vi "assemblies to tables.vi"(11 "assemblies":T1[](array[typedef])) -> (3 "Item Names":string[][](array[string]))   [LabVIEW 2013, in "EthernetIP editor node.lvclass"]
uses:
  EthernetIP editor node.lvclass
  configuration/assembly type.ctl
  configuration/EthernetIP configuration.lvclass
  configuration/assembly definition.ctl
  <vilib>/NI/Tag Bus/tag/Data Type.ctl
  <vilib>/NI/Tag Bus/tag/tag descriptor.lvclass
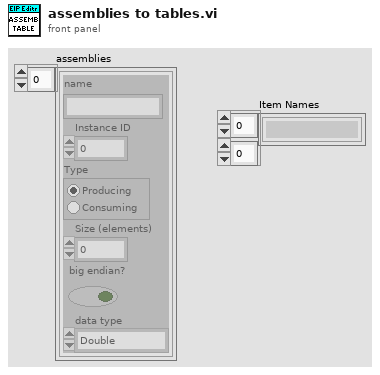
[diagram p1: front panel]
types:
  T1 = typedef "EthernetIP configuration.lvclass/assembly definition.ctl" = cluster{"name":string, "Instance ID":u32, "Type":T2, "Size (elements)":u32, "big endian?":bool, "data type":T3}
  T2 = typedef "EthernetIP configuration.lvclass/assembly type.ctl" = enum32{"Producing", "Consuming"}
  T3 = typedef "tag bus.lvlib/tag descriptor.lvclass/Data Type.ctl" = enum16{"Double", "Single", "I64", "I32", "I16", "I8", "U64", "U32", "U16", "U8", "Boolean", "String", "Array of Double", "Array of Single", "Array of I64", "Array of I32", "Array of I16", "Array of I8", "Array of U64", "Array of U32", "Array of U16", "Array of U8", "Array of Boolean", "Array of String"}
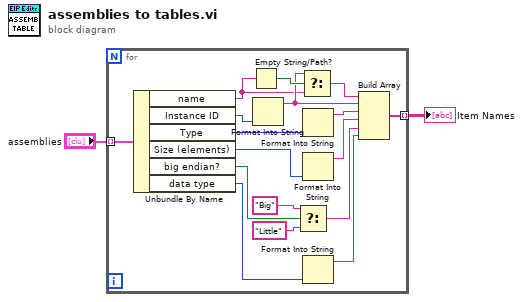
[diagram p0: block diagram]
diagram:
  n1 = for {
    tunnel: "assemblies" -> [w19] mode=indexing
    tunnel: [w13] -> w1 mode=indexing
    n2 = Unbundle By Name(w19) -> ("name"=w9:string, "Instance ID"=w16:u32, "Type"=w17:T2, "Size (elements)"=w18:u32, "big endian?"=w6:bool, "data type"=w4:T3)
    n3 = Empty String/Path?(string/path=w9) -> (empty?=w12:bool)
    n4 = Format Into String(w16) -> (resulting string=w10:string)  [unwired: 3 in, 1 out]
    n5 = Select(t="Big" ("resulting string"), s=w6, f="Little" ("resulting string")) -> (s? t:f=w5:string)
    n6 = Select(t=w10, s=w12, f=w9) -> (s? t:f=w11:string)
    n7 = Format Into String(w17) -> (resulting string=w15:string)  [unwired: 3 in, 1 out]
    n8 = Format Into String(w18) -> (resulting string=w14:string)  [unwired: 3 in, 1 out]
    n9 = Format Into String(w4) -> (resulting string=w3:string)  [unwired: 3 in, 1 out]
    n10 = Build Array(w11, w10, w15, w14, w5, w3) -> (w13:string[])
  }
  "Item Names" <- w1
